vi "Funct acq pre-checks Case C.vi"() -> (3 "Proceed":bool)   [LabVIEW 2020]
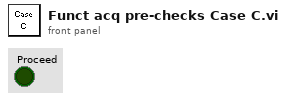
[diagram p1: front panel]
types:
  T1 = typedef "AOL_Globals.ctl" = cluster{"Imaging Protocol":T2, "Number of POI":u16, "Number of Miniscans":u16, "Number of Trials":u16, "Number of Cycles ":u64, "# Averaged Frames":u16, "Laser power (%)":u8, "Pockels (V)":dbl, "Acquisition Length (sec)":dbl, "Fill time (us)":dbl, "POI Dwell time (us)":dbl, "Miniscan Dwell time per pixel (us)":dbl, "PMT 1":dbl, "PMT 2":dbl, "Back Apperture (mA)":dbl, "Frame Size":T3, "Center Frequency":dbl, "Field of View (norm)":dbl, "DwellTime (us)":dbl, "Wavelength (nm)":dbl, "Zoom":dbl, "AOL Z":dbl, "AOL Mode":T4, "GridXY":dbl, "GridZ":dbl, "TriggerPeriod (sec)":dbl, "Number of Pixels in Miniscan":u16, "Experiment folder path":path, "X centre":dbl, "Y centre":dbl, "Angle (degrees)":dbl, "Plane Mode":T5, "Threshold":u16[], "Regenerate Chirps":bool, "Rectangle ROI length (pixels)":u16, "Rectangle ROI height (pixels)":u16, "AOD fill":u16, "StartupDelay":i32, "Samples Wait after Trigger":u16, "Slip Cycle":u32, "Add Cycle":bool, "Functional Mode":T6, "Z Start":dbl, "Z Stop":dbl, "# Planes":i32, "Total Pixels":i32, "Variable Miniscan Pixels":u16[], "Use Variable Length":bool, "Use Variable Resolution":bool, "Laser power (%) at Z Start":u8, "Laser power (%) at Z Stop":u8, "Ref Z Step":i8, "Ref Dwell Time (us)":dbl, "Field of View (um)":dbl}
  T2 = typedef "Imaging Protocols enum.ctl" = enum16{"AOL Z-Stack", "Motor Z Stack", "Functional Acquisition", "Single Plane Acquisition", "Volume Acquisition", "Live Imaging", "Live Plane Imaging", "Live Volume Imaging"}
  T3 = typedef "Frame Size.ctl" = u16
  T4 = typedef "AOL modes.ctl" = enum16{"Raster", "Structural", "Pointing", "Mini Scan", "Alignment"}
  T5 = typedef "Plane Mode.ctl" = u16
  T6 = typedef "Functional Mode.ctl" = enum16{"Point", "Line", "Patch", "Plane", "Volume"}
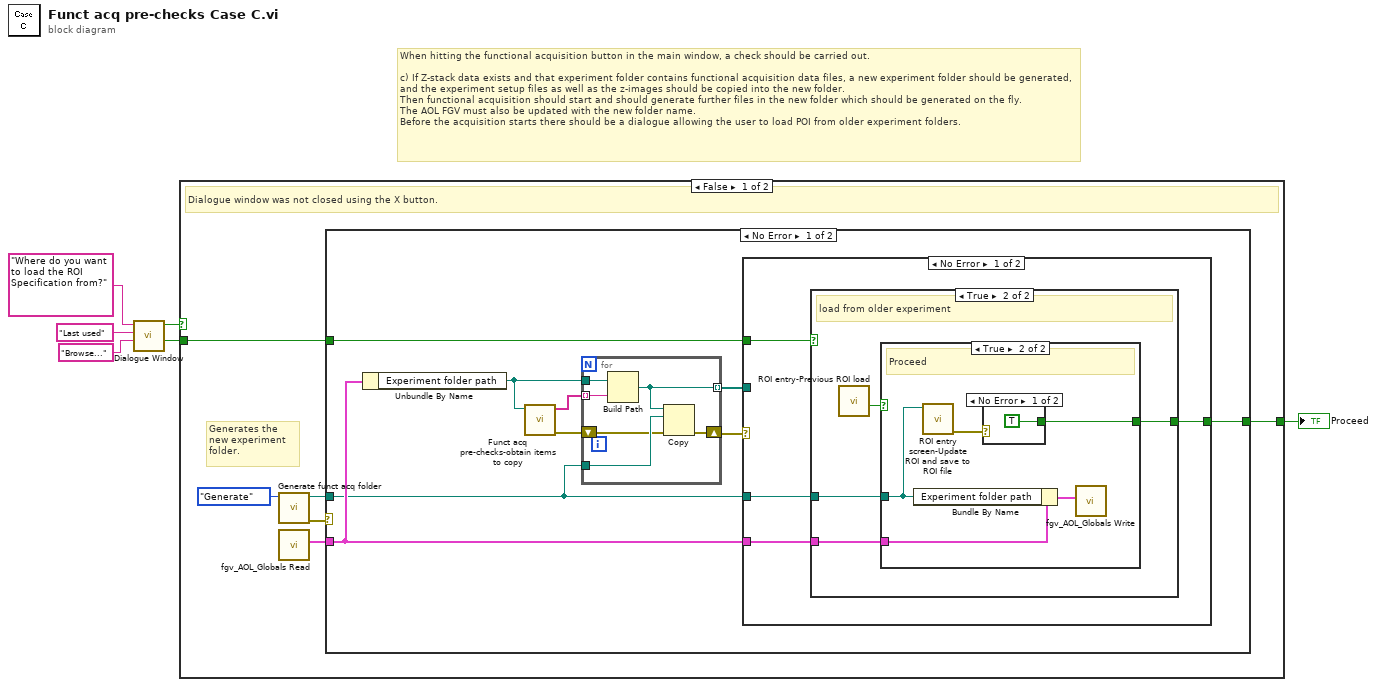
[diagram p0: block diagram]
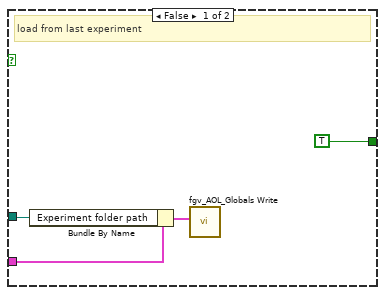
[diagram p2: hidden frame]
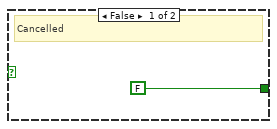
[diagram p3: hidden frame]
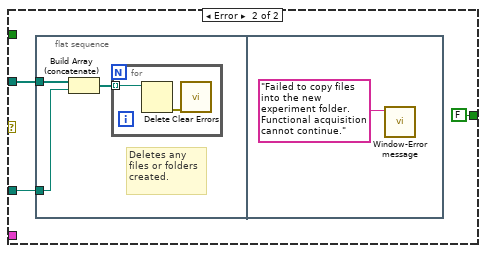
[diagram p5: hidden frame]
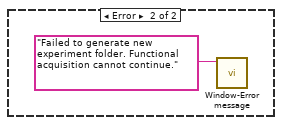
[diagram p6: hidden frame]
diagram:
  # "When hitting the functional acquisition button in the main window, a check should be carried out.\n\nc) If Z-stack data exists and that experiment folder contains functional acquisition data files, a new experiment folder should be generated, and the experiment setup files as well as the z-images should be copied into the new folder. \nThen functional acquisition should start and should generate further files in the new folder which should be generated on the fly. \nThe AOL FGV must also be updated with the new folder name. \nBefore the acquisition starts there should be a dialogue allowing the user to load POI from older experiment folders."
  n1 = call "Dialogue Window.vi"("Caption-Left button (Cancel)"="Browse...", "Caption-Right button (OK)"="Last used", "Message string"="Where do you want to load the ROI Specification from?") -> ("Cancelled (Left button pressed)"=w2:bool, "Panel closed"=w1:bool)  [unwired: 6 in, 1 out]
  n2 = case shown="False" w1 {
    tunnel: [w12 _] -> w6
    tunnel: w2 -> [w11 _]
    frame False {
      # "Generates the new experiment folder."
      # "Dialogue window was not closed using the X button."
      n3 = call "Generate funct acq folder.vi"("Function"=enum16{"Generate", "Obtain"}."Generate") -> ("error out"=w7:errorcluster, "Funct acq experiment folder path"=w8:path)  [unwired: 9 in]
      n4 = call "fgv_AOL_Globals Read.vi"() -> ("AOL_Globals"=w10:T1)  [unwired: 9 in, 2 out]
      n5 = case shown="No Error" w7 {
        tunnel: [w21 _] -> w12
        tunnel: w11 -> [w15 _]
        tunnel: w10 -> [w14 _]
        tunnel: w8 -> [w13 _]
        frame No Error {
          n6 = Unbundle By Name(w14) -> ("Experiment folder path"=w20:path)
          n7 = call "Funct acq pre-checks-obtain items to copy.vi"("Experiment folder path"=w20) -> ("error out"=w19:errorcluster, "Files and folders to copy"=w16:string[])  [unwired: 9 in]
          n8 = for {
            tunnel: w13 -> [w55]
            tunnel: w16 -> [w53] mode=indexing
            tunnel: w20 -> [w54]
            shift-right: [w52] -> w18
            shift-left: w19 -> [w51]
            tunnel: [w50] -> w17 mode=indexing
            n9 = Build Path(base path=w54, name or relative path=w53) -> (appended path=w50:path)
            n10 = Copy(8:w51, 10:w55, 11:w50) -> (0:w52:errorcluster)  [unwired: 2 in, 2 out]
          }
          n11 = case shown="No Error" w18 {
            tunnel: [w25 FALSE] -> w21
            tunnel: w17 -> [_ w42]
            tunnel: w13 -> [w23 w41]
            tunnel: w14 -> [w24 _]
            tunnel: w15 -> [w22 _]
            frame No Error {
              n12 = case shown="True" w22 {
                tunnel: w23 -> [w26 w32]
                tunnel: [TRUE w31] -> w25
                tunnel: w24 -> [w27 w30]
                frame False {
                  # "load from last experiment"
                  n13 = Bundle By Name(cluster=w27, "Experiment folder path"=w26) -> (w28:T1)
                  n14 = call "fgv_AOL_Globals Write.vi"("AOL_Globals"=w28) -> ()  [unwired: 10 in, 1 out]
                }
                frame True {
                  # "load from older experiment"
                  n15 = call "ROI entry-Previous ROI load.vi"() -> ("Proceed"=w33:bool)  [unwired: 11 in]
                  n16 = case shown="True" w33 {
                    tunnel: w32 -> [_ w37]
                    tunnel: [FALSE w39] -> w31
                    tunnel: w30 -> [_ w36]
                    frame False {
                      # "Cancelled"
                    }
                    frame True {
                      # "Proceed"
                      n17 = Bundle By Name(cluster=w36, "Experiment folder path"=w37) -> (w38:T1)
                      n18 = call "ROI entry screen-Update ROI and save to ROI file.vi"("Experiment folder path"=w37) -> ("Error Out"=w35:errorcluster)  [unwired: 9 in, 1 out]
                      n19 = case shown="No Error" w35 {
                        tunnel: [TRUE _] -> w39
                        frame No Error {
                        }
                        frame Error {
                        }
                      }
                      n20 = call "fgv_AOL_Globals Write.vi"("AOL_Globals"=w38) -> ()  [unwired: 10 in, 1 out]
                    }
                  }
                }
              }
            }
            frame Error {
              n21 = flat-sequence {
                tunnel: w42 -> [w46]
                tunnel: w41 -> [w44]
                frame #0 {
                  # "Deletes any files or folders created."
                  n22 = Build Array (concatenate)(w46, w44) -> (w45:path[])
                  n23 = for {
                    tunnel: w45 -> [w48] mode=indexing
                    n24 = Delete(path (use dialog)=w48) -> (error out=w47:errorcluster)  [unwired: 4 in, 2 out]
                    n25 = call <vilib>:"Clear Errors.vi"("error in (no error)"=w47) -> ()  [unwired: 5 in, 2 out]
                  }
                }
                frame #1 {
                  n26 = call "Window-Error message.vi"("Message"="Failed to copy files into the new experiment folder. Functional acquisition cannot continue." ("Error Source")) -> ()  [unwired: 10 in, 1 out]
                }
              }
            }
          }
        }
        frame Error {
          n27 = call "Window-Error message.vi"("Message"="Failed to generate new experiment folder. Functional acquisition cannot continue." ("Error Source")) -> ()  [unwired: 10 in, 1 out]
        }
      }
    }
    frame True {
      # "Dialogue window was closed using the X button."
    }
  }
  "Proceed" <- w6
